vi "String Array to Comma List.vi"(11 "Array":string[](array[string])) -> (3 "String":string)   [LabVIEW 2011]
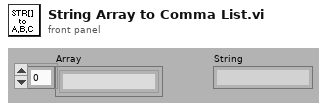
[diagram p1: front panel]
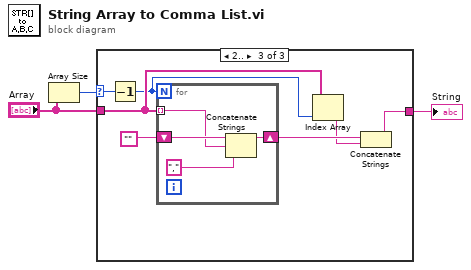
[diagram p0: block diagram]
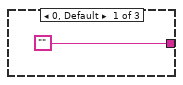
[diagram p2: hidden frame]
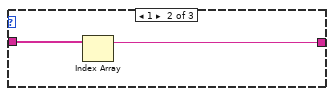
[diagram p3: hidden frame]
diagram:
  n1 = Array Size(array="Array") -> (size(s)=w1:i32)
  n2 = case shown="2.." w1 {
    selector: w1 -> [_ _ w13]
    tunnel: ["" w5 w7] -> w2
    tunnel: "Array" -> [_ w6 w11]
    frame 0, Default {
    }
    frame 1 {
      n3 = Index Array(array=w6) -> (element=w5:string)  [unwired: 1 in]
    }
    frame 2.. {
      n4 = Decrement(x=w13) -> (x-1=w10:i32)
      n5 = for {
        N: w10 -> [_]
        tunnel: w11 -> [w16] mode=indexing
        shift-right: [w15] -> w9
        shift-left: "" -> [w17]
        n6 = Concatenate Strings(w17, w16, ",") -> (w15:string)
      }
      n7 = Index Array(array=w11, index=w10) -> (element=w8:string)
      n8 = Concatenate Strings(w9, w8) -> (w7:string)
    }
  }
  "String" <- w2
